vi "sendValue.vi"(8 "error in (no error)":errorcluster, 10 "data":variant, 11 "azimuthState in":refnum<class "azimuthState.lvclass">) -> (0 "error out":errorcluster, 2 "function return":i32, 3 "azimuthState out":refnum<class "azimuthState.lvclass">)   [LabVIEW 2016, in "SALLV_AtDome_Messaging.lvlib" / "azimuthState.lvclass"]
uses:
  azimuthState.lvclass
  ts_sallv_AtDome/DataTypes/logevent_azimuthState.ctl
  ts_sallv_AtDome/SALLV_AtDome.lvlib
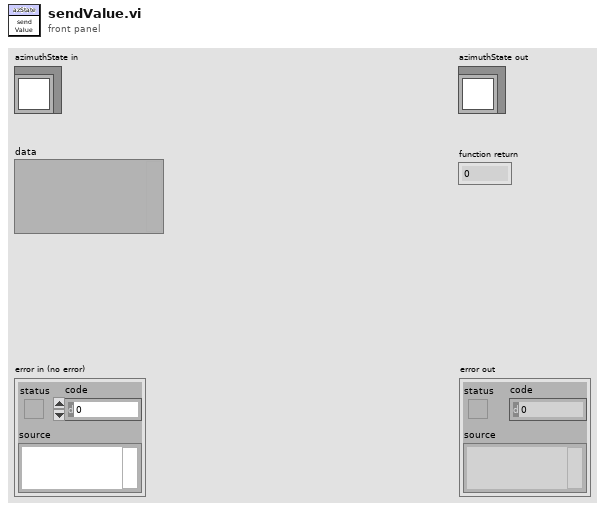
[diagram p1: front panel]
types:
  T1 = typedef "SALLV_AtDome.lvlib/logevent_azimuthState.ctl" = cluster{"state":i32, "priority":i32}
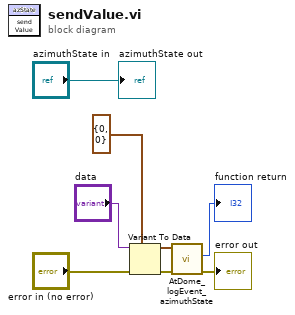
[diagram p0: block diagram]
diagram:
  n1 = Variant To Data(error in="error in (no error)", type=T1 {"state"=0, "priority"=0} ("logevent_azimuthState_Ctl"), Variant="data") -> (data=w4:T1, error out=w5:errorcluster)
  n2 = call "AtDome_logEvent_azimuthState.vi"("error in (no error)"=w5, "logevent_azimuthState_Ctl"=w4) -> ("error out"=→"error out":errorcluster, "function return"=→"function return":i32)  [unwired: 7 in, 1 out]
  "azimuthState out" <- "azimuthState in"
